vi "8.vi"() -> ()   [LabVIEW 2023]
panel:
  out "Waveform Chart":dbl(graph)
  in  "Play Button":bool
  in  "stop":bool
  in  "A":dbl(slide) scale=0.0..100.0
  in  "k":dbl(slide) scale=0.0..10.0
  in  "m":dbl(slide) scale=0.0..10.0
  out "2D Picture":picture
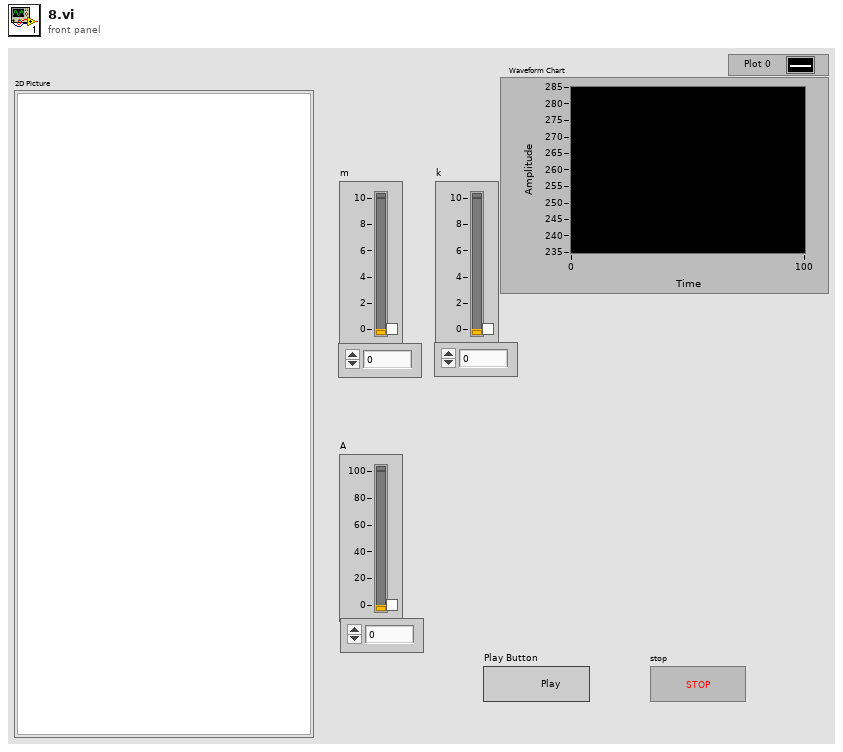
[diagram p1: front panel]
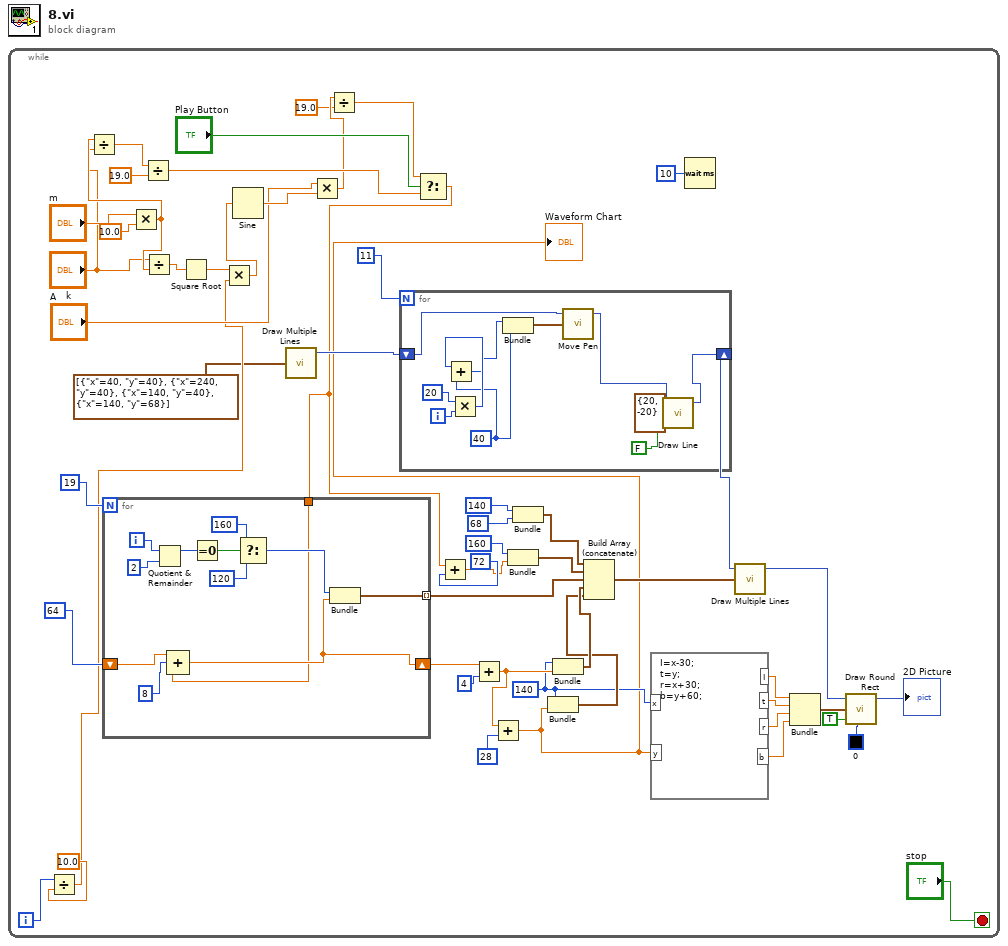
[diagram p0: block diagram]
diagram:
  n1 = while {
    i -> [w16]
    stop <- "stop" stop-if-true
    w30 = 140
    n2 = Divide(x=w16, y=10.0) -> (x/y=w15:dbl)
    n3 = Multiply(x="m", y=10.0) -> (x*y=w12:dbl)
    n4 = Divide(x=w12, y="k") -> (x/y=w10:dbl)
    n5 = Divide(x=w10, y=19.0) -> (x/y=w8:dbl)
    n6 = Divide(x="k", y=w12) -> (x/y=w21:dbl)
    n7 = Square Root(x=w21) -> (sqrt(x)=w20:dbl)
    n8 = Multiply(x=w20, y=w15) -> (x*y=w24:dbl)
    n9 = Sine(x=w24) -> (sin(x)=w23:dbl)
    n10 = call <vilib>:"Draw Multiple Lines.vi"("line endpoints"=cluster{"x":i16, "y":i16}[] [{"x"=40, "y"=40}, {"x"=240, "y"=40}, {"x"=140, "y"=40}, {"x"=140, "y"=68}]) -> ("new picture"=w54:picture)  [unwired: 8 in]
    n11 = Multiply(x="A", y=w23) -> (x*y=w7:dbl)
    n12 = Divide(x=w7, y=19.0) -> (x/y=w5:dbl)
    n13 = for {
      N: 11 -> [_]
      shift-right: [w70] -> w37
      shift-left: w54 -> [w71]
      i -> [w76]
      w73 = 40
      n14 = Multiply(x=20, y=w76) -> (x*y=w74:i32)
      n15 = Add(x=w74, y=w73) -> (x+y=w72:i32)
      n16 = Bundle(w72, w73) -> (w77:cluster{i32, i32})  [unwired: 1 in]
      n17 = call <vilib>:"Move Pen.vi"("new position"=w77, "picture"=w71) -> ("new picture"=w69:picture)  [unwired: 3 in]
      n18 = call <vilib>:"Draw Line.vi"("picture"=w69, "end point"=cluster{"x":i16, "y":i16} {"x"=20, "y"=-20}, "absolute coordinates?(T)"=FALSE ("fill?(F)")) -> ("new picture"=w70:picture)  [unwired: 6 in]
    }
    n19 = Select(t=w5, s="Play Button", f=w8) -> (s? t:f=w4:dbl)
    n20 = for {
      N: 19 -> [_]
      shift-right: [w57] -> w48
      shift-left: 64 -> [w59]
      tunnel: [w56] -> w50 mode=indexing
      tunnel: w4 -> [w55]
      i -> [w66]
      n21 = Quotient & Remainder(x=w66, y=2) -> (x-y*floor(x/y)=w64:i32)  [unwired: 1 out]
      n22 = Compound Arithmetic op=ADD(w59, 8, w55) -> (w57:dbl)
      n23 = Equal To 0?(x=w64) -> (x = 0?=w63:bool)
      n24 = Select(t=160, s=w63, f=120) -> (s? t:f=w60:i32)
      n25 = Bundle(w60, w57) -> (w56:cluster{i32, dbl})  [unwired: 1 in]
    }
    n26 = Add(x=w4, y=72) -> (x+y=w2:dbl)
    n27 = Add(x=w48, y=4) -> (x+y=w46:dbl)
    n28 = Add(x=w46, y=28) -> (x+y=w13:dbl)
    "Waveform Chart" <- w13
    n29 = Bundle(160, w2) -> (w42:cluster{i32, dbl})  [unwired: 1 in]
    n30 = Bundle(140, 68) -> (w39:cluster{i32, i32})  [unwired: 1 in]
    n31 = Bundle(w30, w13) -> (w44:cluster{i32, dbl})  [unwired: 1 in]
    n32 = Bundle(w30, w46) -> (w45:cluster{i32, dbl})  [unwired: 1 in]
    n33 = Build Array (concatenate)(w39, w42, w50, w45, w44) -> (w38:cluster{i32, dbl}[])
    n34 = formula code="I=x-30;\nt=y;\nr=x+30;\nb=y+60;"("x"=w30, "y"=w13) -> ("I"=w36:dbl, "t"=w25:dbl, "r"=w35:dbl, "b"=w34:dbl)
    n35 = Wait (ms)(milliseconds to wait=u32 10) -> ()  [unwired: 1 out]
    n36 = call <vilib>:"Draw Multiple Lines.vi"("picture"=w37, "line endpoints"=w38) -> ("new picture"=w32:picture)  [unwired: 7 in]
    n37 = Bundle("I"=w36, "t"=w25, "r"=w35, "b"=w34) -> (w33:cluster{"I":dbl, "t":dbl, "r":dbl, "b":dbl})  [unwired: 1 in]
    n38 = call <vilib>:"Draw Round Rect.vi"("picture"=w32, "rect"=w33, "fill?(F)"=TRUE, "color(black)"=u32 0) -> ("new picture"=→"2D Picture":picture)  [unwired: 5 in]
  }
